vi "All Stop.vi"(8 "error in (no error)":errorcluster, 11 "PM_Group in":refnum<class "PM_Group.lvclass">) -> (0 "error out":errorcluster, 3 "PM_Group out":refnum<class "PM_Group.lvclass">)   [LabVIEW 2019, in "PM_Group.lvclass"]
uses:
  PM_Group.lvclass
  TypeDef/Motor N.ctl
  TypeDef/Active Motor.ctl
  PM_Group.lvclass/PM_Group.ctl
  Engine_1DO_2DI_class/Engine_1DO_2DI.lvclass
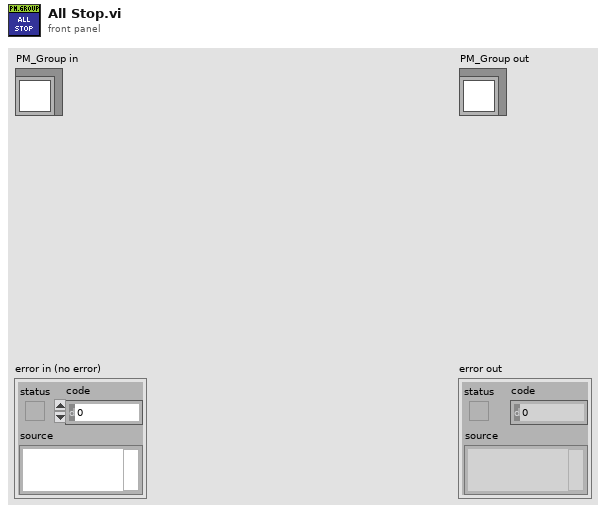
[diagram p1: front panel]
types:
  T1 = typedef "Motor N.ctl" = enum16{"M12", "M21", "M24"}
  T2 = typedef "Active Motor.ctl" = cluster{"Active":bool, "MotorN":T1}
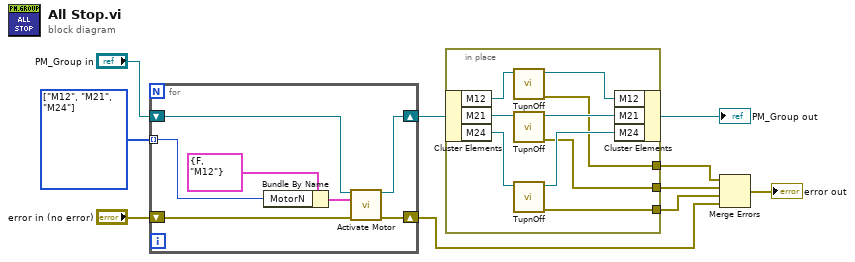
[diagram p0: block diagram]
diagram:
  w8 = T1[] [enum."M12", enum."M21", enum."M24"] items=["M12", "M21", "M24"] ("MotorN")
  n1 = for {
    shift-right: [w16] -> w7
    shift-left: "PM_Group in" -> [w17]
    shift-right: [w14] -> w4
    shift-left: "error in (no error)" -> [w15]
    tunnel: w8 -> [w11] mode=indexing
    n2 = Bundle By Name(cluster=T2 {"Active"=FALSE, "MotorN"=enum."M12"} ("Active Motor"), "MotorN"=w11) -> (w12:T2)
    n3 = call "Activate Motor.vi"("reference in"=w17, "Active Motor"=w12, "error in (no error)"=w15) -> ("reference out"=w16:refnum<class "PM_Group.lvclass">, "error out"=w14:errorcluster)  [unwired: 11 in]
  }
  n4 = in-place {
    in-place-border: [w20] -> w5
    in-place-border: [w19] -> w3
    in-place-border: [w18] -> w2
    n5 = in-place-cluster #1(w7) -> ("M12"=w26:refnum<class "Engine_1DO_2DI.lvclass">, "M21"=w24:refnum<class "Engine_1DO_2DI.lvclass">, "M24"=w22:refnum<class "Engine_1DO_2DI.lvclass">)
    n6 = call "TupnOff.vi"("Pump_1AI_1DO_2DI in"=w26) -> ("error out"=w20:errorcluster, "Pump_1AI_1DO_2DI out"=w25:refnum<class "Engine_1DO_2DI.lvclass">)  [unwired: 9 in]
    n7 = call "TupnOff.vi"("Pump_1AI_1DO_2DI in"=w24) -> ("error out"=w19:errorcluster, "Pump_1AI_1DO_2DI out"=w23:refnum<class "Engine_1DO_2DI.lvclass">)  [unwired: 9 in]
    n8 = call "TupnOff.vi"("Pump_1AI_1DO_2DI in"=w22) -> ("error out"=w18:errorcluster, "Pump_1AI_1DO_2DI out"=w21:refnum<class "Engine_1DO_2DI.lvclass">)  [unwired: 9 in]
    n9 = in-place-cluster #1("M12"=w25, "M21"=w23, "M24"=w21) -> (→"PM_Group out":refnum<class "PM_Group.lvclass">)
  }
  n10 = Merge Errors(w5, w3, w2, w4) -> (→"error out":errorcluster)
